vi "Utility - Configuration File Generator.vi"() -> ()   [LabVIEW 2015]
uses:
  controls/TDMS Properties.ctl
  <vilib>/LabVIEW Targets/FPGA/cRIO/shared/nicrio_ModuleControls/nicrio_cRIO-9234_DataRatesRing2.ctl
  controls/Acquisition and Logging Configuration.ctl
  <vilib>/Utility/xml.llb/Write to XML File(string).vi
panel:
  in  "Date Rate":T1=20 caption="采样率" items=["51.200 kS/s (NI 9234)"=1, "25.600 kS/s (NI 9234)"=2, "17.067 kS/s (NI 9234)"=3, "12.800 kS/s (NI 9234)"=4, "10.240 kS/s (NI 9234)"=5, "8.533 kS/s (NI 9234)"=6, "7.314 kS/s (NI 9234)"=7, "6.400 kS/s (NI 9234)"=8, "5.689 kS/s (NI 9234)"=9, "5.120 kS/s (NI 9234)"=10, "4.654 kS/s (NI 9234)"=11, "4.267 kS/s (NI 9234)"=12, "3.938 kS/s (NI 9234)"=13, "3.657 kS/s (NI 9234)"=14, "3.413 kS/s (NI 9234)"=15, "3.200 kS/s (NI 9234)"=16, "3.012 kS/s (NI 9234)"=17, "2.845 kS/s (NI 9234)"=18, "2.695 kS/s (NI 9234)"=19, "2.560 kS/s (NI 9234)"=20, "2.438 kS/s (NI 9234)"=21, "2.328 kS/s (NI 9234)"=22, "2.226 kS/s (NI 9234)"=23, "2.133 kS/s (NI 9234)"=24, "2.048 kS/s (NI 9234)"=25, "1.969 kS/s (NI 9234)"=26, "1.896 kS/s (NI 9234)"=27, "1.829 kS/s (NI 9234)"=28, "1.765 kS/s (NI 9234)"=29, "1.707 kS/s (NI 9234)"=30, "1.652 kS/s (NI 9234)"=31]
  in  "Data File Name":string="cRIO_Data" caption="数据文件名"
  in  "TDMS Properties":T2[](array[typedef])=[{"Name"="Company", "Value"="TongRui"}, {"Name"="Developer", "Value"="SUN"}] caption="TDMS属性"
  in  "Trigger - Time (Minute)":i32=5 caption="触发－时间（分钟）"
  in  "Trigger - Channel":i32 caption="触发－通道"
  in  "Trigger - RMS Value":dbl=0.9999999999999994 caption="触发－均方根值"
  in  "Channel Names":string[](array[string])=["Mod1\\AI0", "Mod1\\AI1", "Mod1\\AI2", "Mod1\\AI3"] caption="通道名"
  in  "Channel Scale Array":fxp<+,24,12>[](array[numeric])=[1.0, 1.0, 1.0, 1.0] caption="通道换算数组"
  in  "Number of Channels":i32=4 caption="通道数"
  in  "Number of Reads to Save":i32=20 caption="用于保存的读取次数"
  in  "Samples per Read":i32=1280 caption="每次读取采样"
  # "指南：为下列控件赋值，然后运行VI，在项目的根目录中生成Config.xml文件。\n\n注：生成Config.xml以后，需将其复制至RT终端根目录中。"
  # "通道"
  # "保存"
  # "采样"
  # "触发"
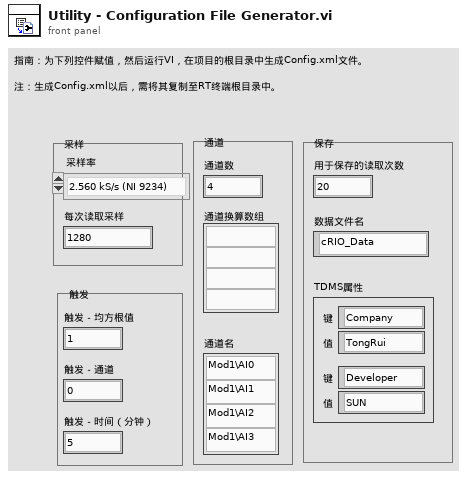
[diagram p1: front panel]
types:
  T1 = typedef "nicrio_cRIO-9234_DataRatesRing2.ctl" = u8
  T2 = typedef "TDMS Properties.ctl" = cluster{"Name":string, "Value":string}
  T3 = typedef "Acquisition and Logging Configuration.ctl" = cluster{"Samples per Read":i32, "Number of Reads to Save":i32, "Number of Channels":i32, "Channel Scale Array":fxp<+,24,12>[], "Channel Names":string[], "Trigger - RMS Value":dbl, "Trigger - Channel":i32, "Trigger - Time (Minute)":i32, "TDMS Properties":T2[], "Data File Name":string, "Date Rate":T1}
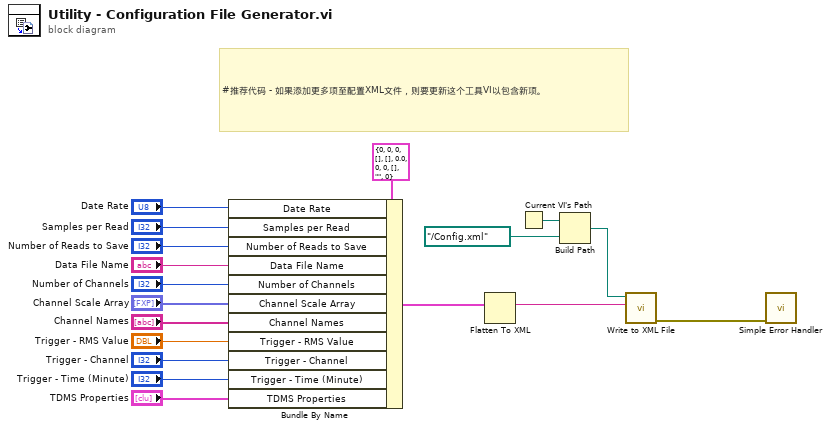
[diagram p0: block diagram]
diagram:
  # "#推荐代码 - 如果添加更多项至配置XML文件，则要更新这个工具VI以包含新项。"
  n1 = Bundle By Name(cluster=T3 {"Samples per Read"=0, "Number of Reads to Save"=0, "Number of Channels"=0, "Channel Scale Array"=[], "Channel Names"=[], "Trigger - RMS Value"=0.0, "Trigger - Channel"=0, "Trigger - Time (Minute)"=0, "TDMS Properties"=[], "Data File Name"="", "Date Rate"=0} ("Acquisition and Logging Configuration"), "Date Rate"="Date Rate", "Samples per Read"="Samples per Read", "Number of Reads to Save"="Number of Reads to Save", "Data File Name"="Data File Name", "Number of Channels"="Number of Channels", "Channel Scale Array"="Channel Scale Array", "Channel Names"="Channel Names", "Trigger - RMS Value"="Trigger - RMS Value", "Trigger - Channel"="Trigger - Channel", "Trigger - Time (Minute)"="Trigger - Time (Minute)", "TDMS Properties"="TDMS Properties") -> (w17:T3)
  n2 = Flatten To XML(anything=w17) -> (xml string=w16:string)
  n3 = Current VI's Path() -> (path=w15:path)
  n4 = Build Path(base path=w15, name or relative path=path "../Config.xml") -> (appended path=w13:path)
  n5 = call-poly <vilib>:"Write to XML File.vi"("XML Input"=w16, "XML File Path"=w13) -> ("error out"=w12:errorcluster)  [unwired: 7 in, 2 out]
  n6 = call <vilib>:"Simple Error Handler.vi"("error in (no error)"=w12) -> ()  [unwired: 4 in, 5 out]
